vi "Load MP3.vi"(8 "error in (no error)":errorcluster, 11 "Path":path) -> (0 "error out":errorcluster, 1 "data":waveform(i16)[](array[waveform]), 2 "Sample Rate (Hz)":i32, 3 "Channels":i32, 5 "Length (Samples)":i32)   [LabVIEW 2018, in "Audio File Input.lvlib"]
doc: "Loads an MP3 file from disk.\n\n<b>Priority:</b> Background priority (lowest)"
uses:
  Audio File Input.lvlib
  external/minimp3_wrapper/minimp3_wrapper.dll
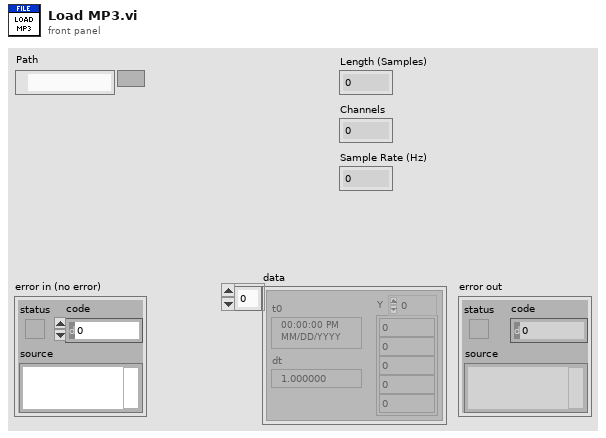
[diagram p1: front panel]
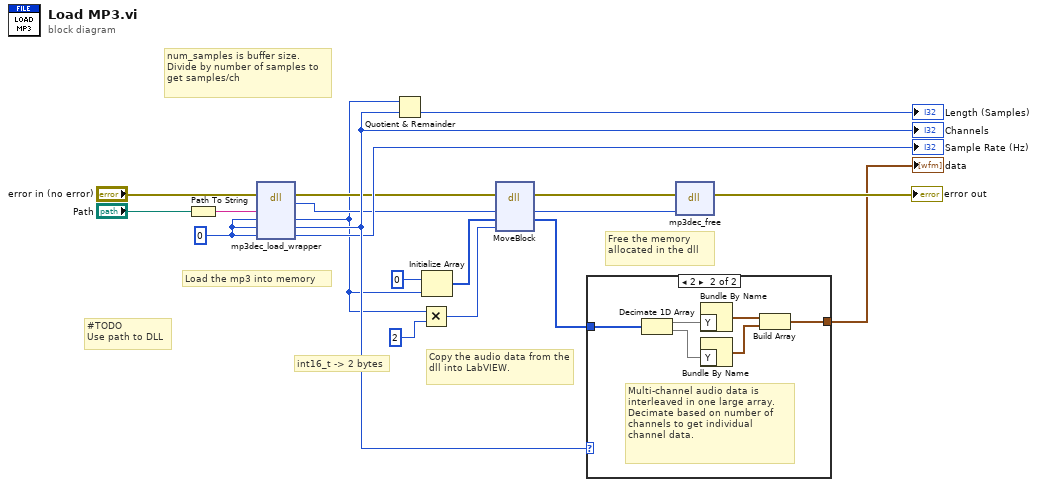
[diagram p0: block diagram]
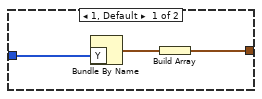
[diagram p2: hidden frame]
diagram:
  w11 = 0 ("num_samples")
  # "#TODO\nUse path to DLL"
  # "num_samples is buffer size. Divide by number of samples to get samples/ch"
  # "Free the memory allocated in the dll"
  # "Copy the audio data from the dll into LabVIEW."
  # "Load the mp3 into memory"
  # "int16_t -> 2 bytes"
  n1 = Path To String(path="Path") -> (string=w12:string)
  n2 = dll-call lib="C:/github/dataflowg/dataflow-dj/external/minimp3_wrapper/minimp3_wrapper.dll" fn="mp3dec_load_wrapper"(error in="error in (no error)", "file_name"=w12, "num_samples"=w11, "channels"=w11, "frequency"=w11) -> (error out=w7:errorcluster, "return type"=w9:i64, "num_samples"=w2:i32, "channels"=w15:i32, "frequency"=→"Sample Rate (Hz)":i32)  [unwired: 3 in, 1 out]
  "Channels" <- w15
  n3 = Quotient & Remainder(x=w2, y=w15) -> (floor(x/y)=→"Length (Samples)":i32)  [unwired: 1 out]
  n4 = Multiply(x=w2, y=2) -> (x*y=w5:i32)
  n5 = Initialize Array(i16 0 ("num_samples"), w2) -> (w8:i16[])
  n6 = dll-call lib="LabVIEW" fn="MoveBlock"(error in=w7, "Address (Pointer)"=w9, "Destination"=w8, "Size"=w5) -> (error out=w3:errorcluster, "Address (Pointer)"=w4:i64, "Destination"=w1:i16[])  [unwired: 4 in, 1 out]
  n7 = case shown="2" w15 {
    tunnel: w1 -> [w22 w28]
    tunnel: [w21 w23] -> w13
    frame 1, Default {
      n8 = Bundle By Name("Y"=w22) -> (w20:waveform(i16))  [unwired: 1 in]
      n9 = Build Array(w20) -> (w21:waveform(i16)[])
    }
    frame 2 {
      # "Multi-channel audio data is interleaved in one large array. Decimate based on number of channels to get individual channel data."
      n10 = Decimate 1D Array(w28) -> (w27:i16[], w26:i16[])
      n11 = Bundle By Name("Y"=w27) -> (w25:waveform(i16))  [unwired: 1 in]
      n12 = Bundle By Name("Y"=w26) -> (w24:waveform(i16))  [unwired: 1 in]
      n13 = Build Array(w25, w24) -> (w23:waveform(i16)[])
    }
  }
  "data" <- w13
  n14 = dll-call lib="C:/github/dataflowg/dataflow-dj/external/minimp3_wrapper/minimp3_wrapper.dll" fn="mp3dec_free"(error in=w3, "Address (Pointer)"=w4) -> (error out=→"error out":errorcluster)  [unwired: 4 in, 1 out]
